vi "Write CFG File.vi"(8 "error in (no error)":errorcluster, 10 "File path":path, 11 "Common Measurements Interface in":refnum<class "Common Measurements Interface.lvclass">) -> (0 "error out":errorcluster, 2 "Section":string, 3 "Common Measurements Interface out":refnum<class "Common Measurements Interface.lvclass">)   [LabVIEW 2015, in "Common Measurements Interface.lvclass"]
uses:
  Common Measurements Interface.lvclass
  Common Measurements Interface.lvclass/Common Measurements Interface.ctl
  Queued Listbox/Queued Listbox.xctl
  Read Measurements Menu.vi
  Mag Lab Measure Interface/Interface with menu/Interface with menu.lvclass
  <vilib>/Utility/config.llb/NI_LVConfig.lvlib
  Mag Lab Error Handler/Mag Lab Error Handler.lvclass
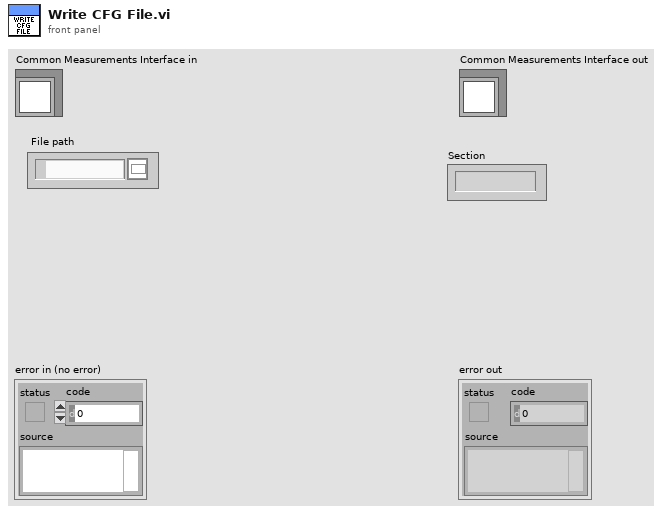
[diagram p1: front panel]
types:
  T1 = typedef "NI_LVConfig.lvlib/Config Data RefNum.ctl" = refnum<k1>
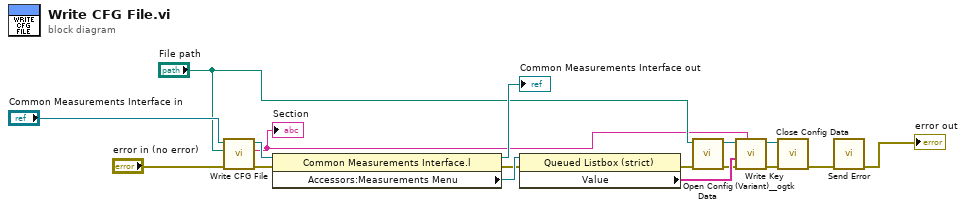
[diagram p0: block diagram]
diagram:
  n1 = call-parent "Write CFG File.vi"("error in (no error)"="error in (no error)", "File path"="File path", "Mag Lab Root in"="Common Measurements Interface in") -> ("error out"=w11:errorcluster, "Section"=w7:string, "Mag Lab Root out"=w17:refnum<class "Common Measurements Interface.lvclass">)  [unwired: 6 in]
  "Section" <- w7
  n2 = property class="Common Measurements Interface.l"(reference=w17, error in=w11) -> (reference out=→"Common Measurements Interface out":refnum<class "Common Measurements Interface.lvclass">, error out=w12:errorcluster, "Accessors:Measurements Menu"=w13:refnum<vi>)
  n3 = property class="Queued Listbox (strict)"(reference=w13, error in=w12) -> (error out=w9:errorcluster, "Value"=w6:string[])  [unwired: 1 out]
  n4 = call <vilib>:"Open Config Data.vi"("error in (no error)"=w9, "configuration file path"="File path") -> ("error out"=w5:errorcluster, "refnum"=w8:T1)  [unwired: 7 in, 1 out]
  n5 = call <userlib>:"Write Key (Variant)__ogtk.vi"("section"=w7, "error in (no error)"=w5, "key-value"=w6, "refnum"=w8) -> ("error out"=w4:errorcluster, "refnum out"=w3:T1)  [unwired: 6 in]
  n6 = call <vilib>:"Close Config Data.vi"("error in (no error)"=w4, "refnum"=w3) -> ("error out"=w2:errorcluster)  [unwired: 8 in, 1 out]
  n7 = call "Send Error.vi"("error in (no error)"=w2) -> ("error out"=→"error out":errorcluster)  [unwired: 9 in, 1 out]
